vi "PopUp.vi"(8 "error in (no error)":errorcluster, 11 "TestBench in":refnum<class "TestBench.lvclass">) -> (0 "error out":errorcluster, 3 "TestBench out":refnum<class "TestBench.lvclass">)   [LabVIEW 2019, in "TestBench.lvlib" / "TestBench.lvclass"]
uses:
  TestBench.lvclass
  TestBench.lvclass/TestBench.ctl
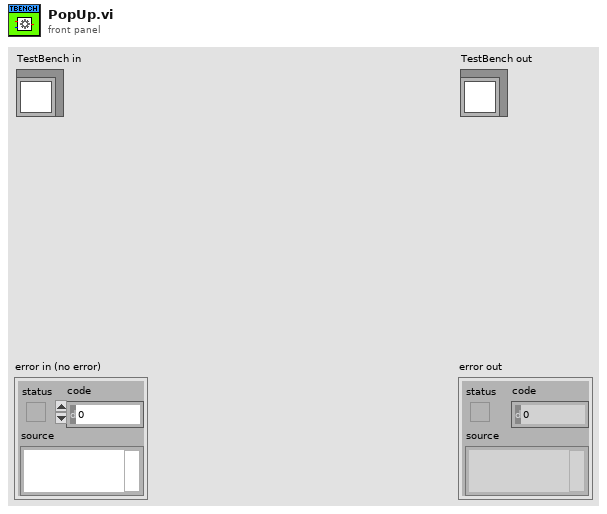
[diagram p1: front panel]
types:
  T1 = enum32{"Invalid", "Standard", "Closed", "Hidden", "Minimized", "Maximized"}
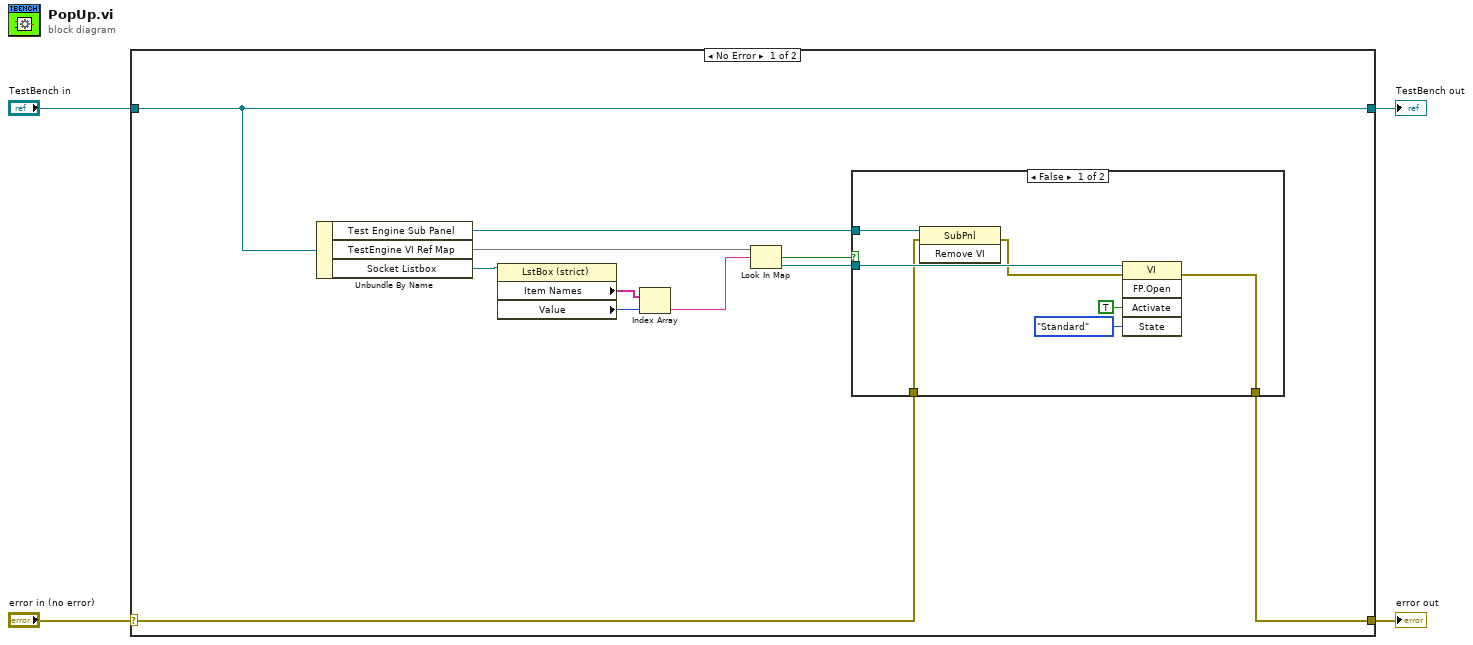
[diagram p0: block diagram]
diagram:
  n1 = case shown="No Error" "error in (no error)" {
    selector: "error in (no error)" -> [w7 w25]
    tunnel: [w6 w25] -> w3
    tunnel: [w15 w24] -> w1
    tunnel: "TestBench in" -> [w15 w24]
    frame No Error {
      n2 = Unbundle By Name(w15) -> ("Test Engine Sub Panel"=w14:refnum<vi>, "TestEngine VI Ref Map"=w10:map{string, refnum<vi>}, "Socket Listbox"=w13:refnum<vi>)
      n3 = property class="LstBox (strict)"(reference=w13) -> ("Item Names"=w11:string[], "Value"=w12:i32)  [unwired: 1 in, 2 out]
      n4 = Index Array(array=w11, index=w12) -> (element=w9:string)
      n5 = Look In Map(map=w10, key=w9) -> (key not found?=w5:bool, value=w8:refnum<vi>)  [unwired: 1 in]
      n6 = case shown="False" w5 {
        tunnel: w14 -> [w22 _]
        tunnel: w8 -> [w21 _]
        tunnel: w7 -> [w17 w23]
        tunnel: [w16 w23] -> w6
        frame False {
          n7 = invoke class="SubPnl" method="Remove VI"(reference=w22, error in=w17) -> (error out=w20:errorcluster)  [unwired: 1 in, 2 out]
          n8 = invoke class="VI" method="FP.Open"(reference=w21, error in=w20, "Activate"=TRUE ("Activate?"), "State"=T1."Standard") -> (error out=w16:errorcluster)  [unwired: 1 in, 4 out]
        }
        frame True {
        }
      }
    }
    frame Error {
    }
  }
  "error out" <- w3
  "TestBench out" <- w1
